vi "Link Async Parameters.vi"(7 "Parameter R Table":refnum<class "Registry.lvclass">, 8 "error in (no error)":errorcluster, 9 "Async Payload":T1 {"Trigger Command" format="%04x"; "Data" format="%04x"; "Data Address" format="%04x"; "Configuration" format="%04x"; "Configuration Address" format="%04x"}, 10 "Parameter W Table":refnum<class "Registry.lvclass">, 11 "Async Message in":refnum<class "Async Message.lvclass">) -> (0 "error out":errorcluster, 2 "Parameter W Table out":refnum<class "Registry.lvclass">, 3 "Async Message out":refnum<class "Async Message.lvclass">, 5 "Parameter R Table out":refnum<class "Registry.lvclass">)   [LabVIEW 2020, in "BCI-1553 API.lvlib" / "Async Message.lvclass"]
doc: "<DO NOT CALL>\n\nCopies the parameters stored in the asynchronous Message to the parameter read or write tables. If the async Message is a transmit command, the read table will be updated. If the async Message is a receive command, the write table will be updated."
uses:
  Async Message.lvclass
  Dependencies/Registry/Registry.lvclass
  TypeDefs/Async Payload.ctl
  Async Message.lvclass/Async Message.ctl
  Dependencies/Registry/Registry.lvclass/Registry.ctl
  BCI-1553 API.lvlib
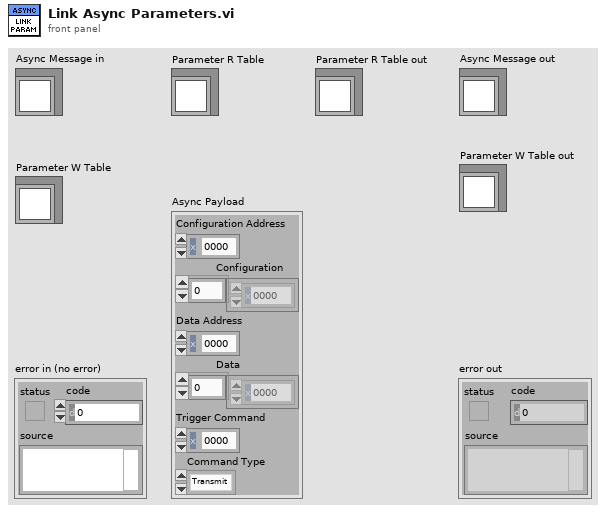
[diagram p1: front panel]
types:
  T1 = typedef "BCI-1553 API.lvlib/Async Payload.ctl" = cluster{"Configuration Address":u16, "Configuration":u16[], "Data Address":u16, "Data":u16[], "Trigger Command":u16, "Command Type":enum16{"Transmit", "Receive"}}
  T2 = typedef "BCI-1553 API.lvlib/Parameter Table Data.ctl" = cluster{"Parameter Name":string, "Base Word":u16, "Address":u16, "Value":u64, "Mask":u16[], "Scaling Info":T3}
  T3 = typedef "BCI-1553 API.lvlib/Scaling Information.ctl" = cluster{"Bit Offset":i32, "Bit Count":i32, "LSB Resolution":dbl, "2's Complement":bool, "Big Endian":bool, "Sign Bit":bool}
  T4 = typedef "BCI-1553 API.lvlib/Command Type.ctl" = enum16{"Transmit", "Receive"}
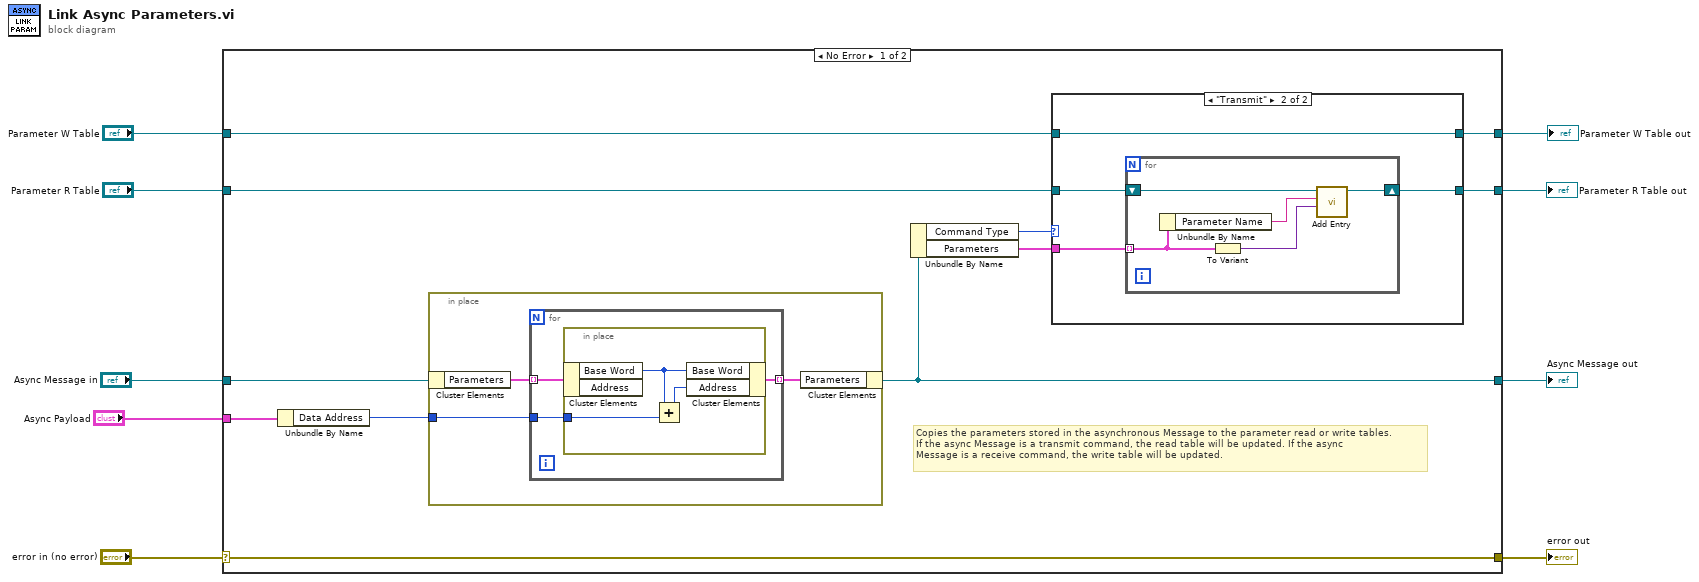
[diagram p0: block diagram]
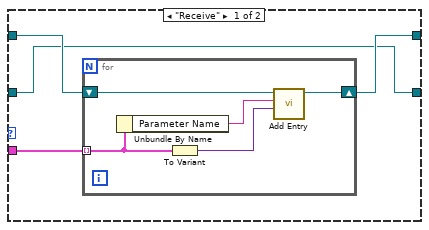
[diagram p2: hidden frame]
diagram:
  n1 = case shown="No Error" "error in (no error)" {
    selector: "error in (no error)" -> [w20 w51]
    tunnel: [w20 w51] -> w8
    tunnel: [w17 w50] -> w6
    tunnel: "Async Message in" -> [w19 w50]
    tunnel: [w15 w48] -> w5
    tunnel: "Parameter R Table" -> [w16 w48]
    tunnel: "Async Payload" -> [w18 _]
    tunnel: "Parameter W Table" -> [w12 w49]
    tunnel: [w11 w49] -> w1
    frame No Error {
      # "Copies the parameters stored in the asynchronous Message to the parameter read or write tables.\nIf the async Message is a transmit command, the read table will be updated. If the async\nMessage is a receive command, the write table will be updated."
      n2 = Unbundle By Name(w18) -> ("Data Address"=w10:u16)
      n3 = in-place {
        in-place-border: w10 -> [w40]
        n4 = in-place-cluster #1(w19) -> ("Parameters"=w41:T2[])
        n5 = for {
          tunnel: w41 -> [w44] mode=indexing
          tunnel: w40 -> [w43]
          tunnel: [w42] -> w39 mode=indexing
          n6 = in-place {
            in-place-border: w43 -> [w47]
            n7 = in-place-cluster #2(w44) -> ("Base Word"=w45:u16)  [unwired: 1 out]
            n8 = Add(x=w45, y=w47) -> (x+y=w46:u16)
            n9 = in-place-cluster #2("Base Word"=w45, "Address"=w46) -> (w42:T2)
          }
        }
        n10 = in-place-cluster #1("Parameters"=w39) -> (w17:refnum<class "Async Message.lvclass">)
      }
      n11 = Unbundle By Name(w17) -> ("Command Type"=w14:T4, "Parameters"=w13:T2[])
      n12 = case shown="\"Transmit\"" w14 {
        tunnel: w16 -> [w21 w32]
        tunnel: [w21 w31] -> w15
        tunnel: w13 -> [w24 w33]
        tunnel: w12 -> [w23 w30]
        tunnel: [w22 w30] -> w11
        frame "Receive" {
          n13 = for {
            shift-right: [w28] -> w22
            shift-left: w23 -> [w29]
            tunnel: w24 -> [w27] mode=indexing
            n14 = Unbundle By Name(w27) -> ("Parameter Name"=w25:string)
            n15 = To Variant(anything=w27) -> (Variant=w26:variant)
            n16 = call "Add Entry.vi"("Value"=w26, "Key"=w25, "Registry in"=w29) -> ("Registry out"=w28:refnum<class "Registry.lvclass">)  [unwired: 6 in, 2 out]
          }
        }
        frame "Transmit" {
          n17 = for {
            shift-right: [w37] -> w31
            shift-left: w32 -> [w38]
            tunnel: w33 -> [w36] mode=indexing
            n18 = Unbundle By Name(w36) -> ("Parameter Name"=w34:string)
            n19 = To Variant(anything=w36) -> (Variant=w35:variant)
            n20 = call "Add Entry.vi"("Value"=w35, "Key"=w34, "Registry in"=w38) -> ("Registry out"=w37:refnum<class "Registry.lvclass">)  [unwired: 6 in, 2 out]
          }
        }
      }
    }
    frame Error {
    }
  }
  "error out" <- w8
  "Async Message out" <- w6
  "Parameter R Table out" <- w5
  "Parameter W Table out" <- w1
